vi "Log Sequence.vi"() -> ()   [LabVIEW 2020, in "LogKonfig.lvlib"]
uses:
  LogKonfig.lvlib
  Visualisierungs Elemente/Button.ctl
  FT-IR/FGV FT-IR Gasliste Aktionen.ctl
  Log Sequence FGV Aktion.ctl
  Allgemein/allgemeine Sub-VIs.lvlib
  FT-IR/FT-IR.lvlib
panel:
  in  "Spektrum File Name":bool caption="Spektrum Datei Name"
  in  "Stopp":T1
  in  "Alle Übernehmen":T1
  in  "Alle Löschen":T1
  in  "Löschen":T1
  in  "Übernehmen":T1
  in  "Original Liste":i32(listbox)
  in  "Konfigurierte Liste":i32(listbox)
  # "Log Reihenfolge"
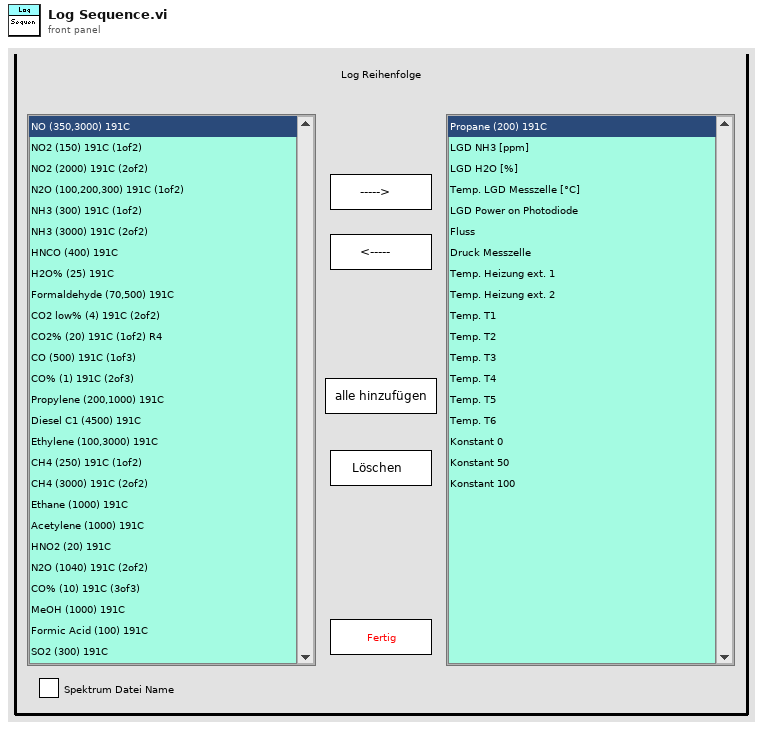
[diagram p1: front panel]
types:
  T1 = typedef "Button.ctl" = bool
  T2 = typedef "LogKonfig.lvlib/Log Sequence FGV Aktion.ctl" = enum16{"initialisieren", "lesen", "schreiben", "laden", "speichern", "übertragen"}
  T3 = typedef "FT-IR.lvlib/FGV FT-IR Gasliste Aktionen.ctl" = enum16{"lesen", "Gasliste FT-IR", "Gasliste ausgelesen", "laden", "speichern", "löschen"}
  T4 = cluster{"Index Array":i32[], "Namen Array":string[], "Spektrum File Name":bool}
  T5 = typedef "String - Ausgabefeld.ctl" = string
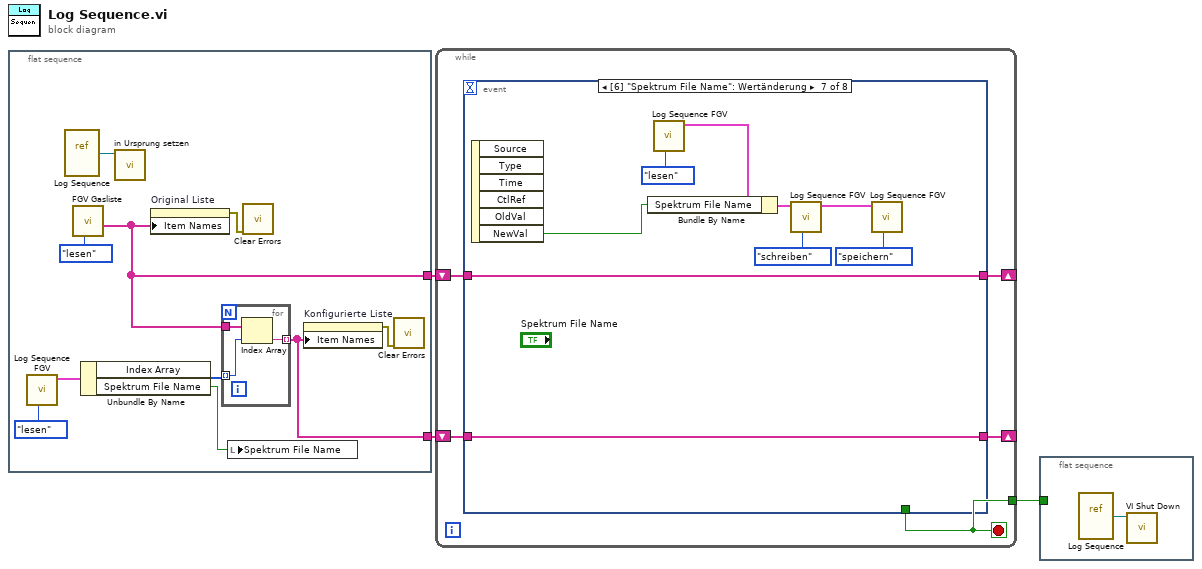
[diagram p0: block diagram]
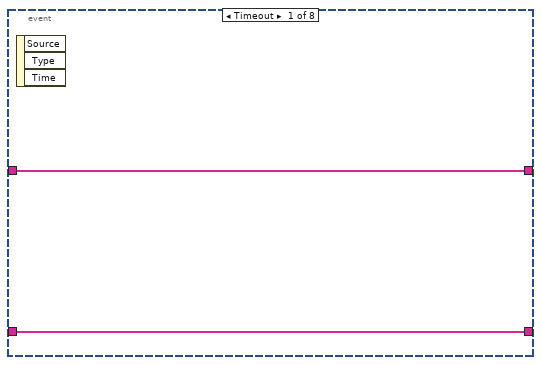
[diagram p2: hidden frame]
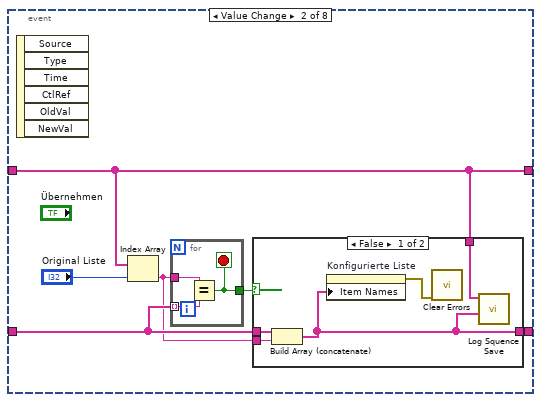
[diagram p3: hidden frame]
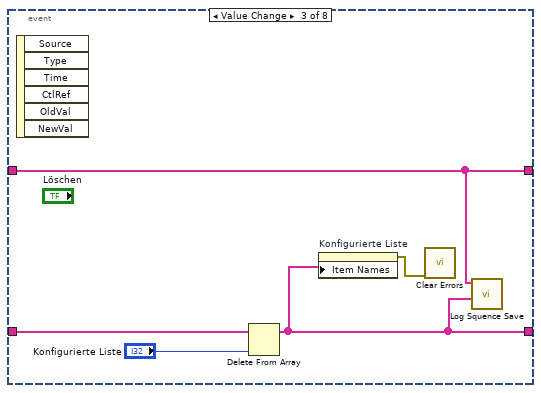
[diagram p5: hidden frame]
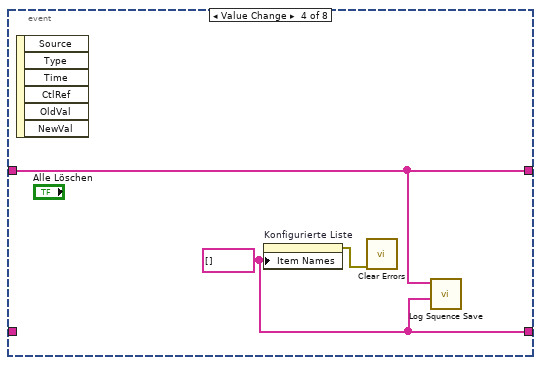
[diagram p6: hidden frame]
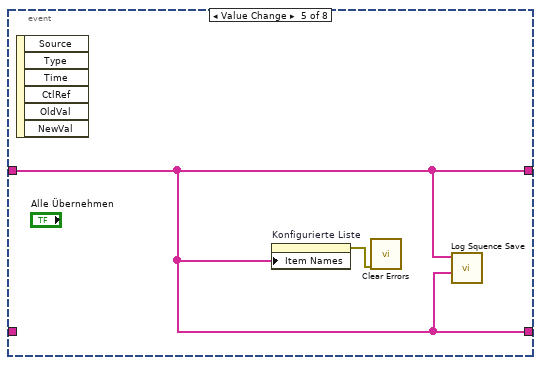
[diagram p7: hidden frame]
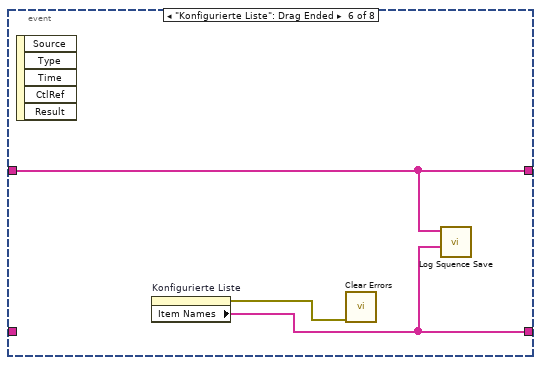
[diagram p8: hidden frame]
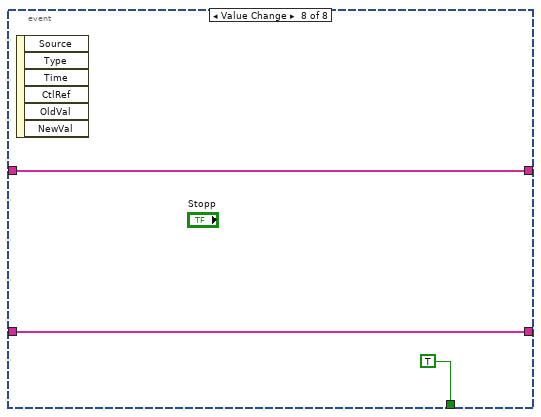
[diagram p9: hidden frame]
diagram:
  n1 = flat-sequence {
    tunnel: [w7] -> w2
    tunnel: [w5] -> w1
    frame #0 {
      n2 = call "Log Sequence FGV.vi"("Aktion"=Log_Sequence_FGV_Aktion."lesen") -> ("Cluster (out)"=w9:T4)  [unwired: 10 in]
      n3 = vi-ref "Log Sequence.vi"() -> (w13:refnum<vi>)
      n4 = call "FGV Gasliste.vi"("Aktionen"=FGV_FT-IR_Gasliste_Aktionen."lesen") -> ("Aktuelle Gasliste gesamt"=w7:T5[])  [unwired: 8 in, 2 out]
      n5 = Unbundle By Name(w9) -> ("Index Array"=w8:i32[], "Spektrum File Name"=w4:bool)
      n6 = call "in Ursprung setzen.vi"("VI Referenz"=w13) -> ()  [unwired: 11 in]
      n7 = property on="Original Liste" class="Listenfeld (strikt)"("Item Names"=w7) -> (error out=w11:errorcluster)  [unwired: 2 in, 1 out]
      n8 = for {
        tunnel: w8 -> [w16] mode=indexing
        tunnel: w7 -> [w15]
        tunnel: [w14] -> w5 mode=indexing
        n9 = Index Array(array=w15, index=w16) -> (element=w14:T5)
      }
      n10 = local write "Spektrum File Name"(w4) -> ()
      n11 = call <vilib>:"Clear Errors.vi"("error in (no error)"=w11) -> ()  [unwired: 5 in, 2 out]
      n12 = property on="Konfigurierte Liste" class="Listenfeld (strikt)"("Item Names"=w5) -> (error out=w6:errorcluster)  [unwired: 2 in, 1 out]
      n13 = call <vilib>:"Clear Errors.vi"("error in (no error)"=w6) -> ()  [unwired: 5 in, 2 out]
    }
  }
  n14 = while {
    tunnel: [w21] -> w3
    shift-right: [w19] -> _
    shift-left: w2 -> [w20]
    shift-right: [w17] -> _
    shift-left: w1 -> [w18]
    stop <- w21 stop-if-true
    n15 = event shown="[6] \"Spektrum File Name\": Wertänderung" {
      selector: _ -> [_ _ _ _ _ _ _ _]
      dyn-events: _ -> [_ _ _ _ _ _ _ _]
      timeout: _ -> [_ _ _ _ _ _ _ _]
      tunnel: [_ _ _ _ _ _ _ TRUE] -> w21
      tunnel: w20 -> [w23 w24 w39 w44 w47 w50 w60 w62]
      tunnel: [w23 w24 w39 w44 w47 w50 w60 w62] -> w19
      tunnel: w18 -> [w22 w27 w43 _ _ _ w59 w61]
      tunnel: [w22 w26 w40 w45 w47 w49 w59 w61] -> w17
      event Timeout {
        n16 = event-data() -> ()  [unwired: 1 in, 3 out]
      }
      event Value Change {
        n17 = event-data() -> ()  [unwired: 1 in, 6 out]
        n18 = Index Array(array=w24, index="Original Liste") -> (element=w25:T5)
        n19 = for {
          tunnel: w25 -> [w38]
          tunnel: w27 -> [w37] mode=indexing
          tunnel: [w36] -> w28
          stop <- w36 stop-if-true
          n20 = Equal?(x=w38, y=w37) -> (x = y?=w36:bool)
        }
        n21 = case shown="False" w28 {
          tunnel: w27 -> [w33 w35]
          tunnel: [w31 w35] -> w26
          tunnel: w25 -> [w32 _]
          tunnel: w24 -> [w30 _]
          frame False {
            n22 = Build Array (concatenate)(w33, w32) -> (w31:T5[])
            n23 = property on="Konfigurierte Liste" class="Listenfeld (strikt)"("Item Names"=w31) -> (error out=w34:errorcluster)  [unwired: 2 in, 1 out]
            n24 = call <vilib>:"Clear Errors.vi"("error in (no error)"=w34) -> ()  [unwired: 5 in, 2 out]
            n25 = call "Log Squence Save.vi"("Item Names"=w31, "Aktuelle Gasliste gesamt"=w30) -> ()  [unwired: 9 in, 1 out]
          }
          frame True {
          }
        }
      }
      event Value Change {
        n26 = event-data() -> ()  [unwired: 1 in, 6 out]
        n27 = Delete From Array(array=w43, index="Konfigurierte Liste") -> (array with subset deleted=w40:T5[])  [unwired: 1 in, 1 out]
        n28 = property on="Konfigurierte Liste" class="Listenfeld (strikt)"("Item Names"=w40) -> (error out=w42:errorcluster)  [unwired: 2 in, 1 out]
        n29 = call <vilib>:"Clear Errors.vi"("error in (no error)"=w42) -> ()  [unwired: 5 in, 2 out]
        n30 = call "Log Squence Save.vi"("Item Names"=w40, "Aktuelle Gasliste gesamt"=w39) -> ()  [unwired: 9 in, 1 out]
      }
      event Value Change {
        w45 = string[] [] ("Objektnamen")
        n31 = event-data() -> ()  [unwired: 1 in, 6 out]
        n32 = property on="Konfigurierte Liste" class="Listenfeld (strikt)"("Item Names"=w45) -> (error out=w46:errorcluster)  [unwired: 2 in, 1 out]
        n33 = call <vilib>:"Clear Errors.vi"("error in (no error)"=w46) -> ()  [unwired: 5 in, 2 out]
        n34 = call "Log Squence Save.vi"("Item Names"=w45, "Aktuelle Gasliste gesamt"=w44) -> ()  [unwired: 9 in, 1 out]
      }
      event Value Change {
        n35 = event-data() -> ()  [unwired: 1 in, 6 out]
        n36 = property on="Konfigurierte Liste" class="Listenfeld (strikt)"("Item Names"=w47) -> (error out=w48:errorcluster)  [unwired: 2 in, 1 out]
        n37 = call <vilib>:"Clear Errors.vi"("error in (no error)"=w48) -> ()  [unwired: 5 in, 2 out]
        n38 = call "Log Squence Save.vi"("Item Names"=w47, "Aktuelle Gasliste gesamt"=w47) -> ()  [unwired: 9 in, 1 out]
      }
      event "Konfigurierte Liste": Drag Ended {
        n39 = event-data() -> ()  [unwired: 1 in, 5 out]
        n40 = property on="Konfigurierte Liste" class="Listenfeld (strikt)"() -> (error out=w51:errorcluster, "Item Names"=w49:string[])  [unwired: 2 in, 1 out]
        n41 = call <vilib>:"Clear Errors.vi"("error in (no error)"=w51) -> ()  [unwired: 5 in, 2 out]
        n42 = call "Log Squence Save.vi"("Item Names"=w49, "Aktuelle Gasliste gesamt"=w50) -> ()  [unwired: 9 in, 1 out]
      }
      event "Spektrum File Name": Value Change {
        n43 = event-data() -> ("NewVal"=w52:bool)  [unwired: 1 in, 5 out]
        n44 = call "Log Sequence FGV.vi"("Aktion"=Log_Sequence_FGV_Aktion."lesen") -> ("Cluster (out)"=w53:T4)  [unwired: 10 in]
        n45 = Bundle By Name(cluster=w53, "Spektrum File Name"=w52) -> (w58:T4)
        n46 = call "Log Sequence FGV.vi"("Aktion"=Log_Sequence_FGV_Aktion."schreiben", "Cluster (in)"=w58) -> ("Cluster (out)"=w55:T4)  [unwired: 9 in]
        n47 = call "Log Sequence FGV.vi"("Aktion"=Log_Sequence_FGV_Aktion."speichern", "Cluster (in)"=w55) -> ()  [unwired: 9 in, 1 out]
      }
      event Value Change {
        n48 = event-data() -> ()  [unwired: 1 in, 6 out]
      }
    }
  }
  n49 = flat-sequence {
    tunnel: w3 -> [_]
    frame #0 {
      n50 = vi-ref "Log Sequence.vi"() -> (w64:refnum<vi>)
      n51 = call "VI Shut Down.vi"("VI Referenz"=w64) -> ()  [unwired: 11 in]
    }
  }
